vi "GFITS_ExecPreImg.vi"(8 "error in (no error)":errorcluster, 10 "preimg":string="none") -> (0 "error out":errorcluster)   [LabVIEW 2016]
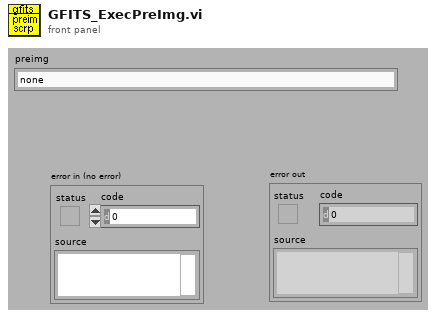
[diagram p1: front panel]
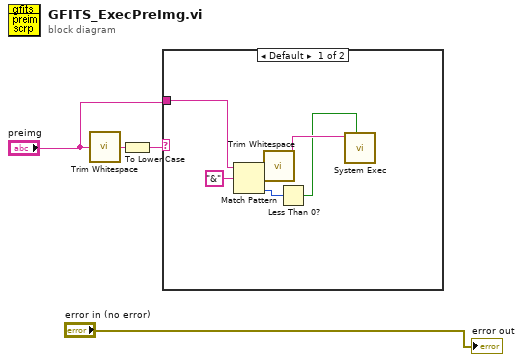
[diagram p0: block diagram]
diagram:
  n1 = call <vilib>:"Trim Whitespace.vi"("string"="preimg") -> ("trimmed string"=w4:string)  [unwired: 1 in]
  n2 = To Lower Case(string=w4) -> (all lower case string=w3:string)
  n3 = case shown="Default" w3 {
    tunnel: "preimg" -> [w10 _]
    frame Default {
      n4 = Match Pattern(string=w10, regular expression="&") -> (before substring=w7:string, offset past match=w8:i32)  [unwired: 3 out]
      n5 = call <vilib>:"Trim Whitespace.vi"("string"=w7) -> ("trimmed string"=w6:string)  [unwired: 1 in]
      n6 = Less Than 0?(x=w8) -> (x < 0?=w5:bool)
      n7 = call <vilib>:"System Exec.vi"("wait until completion? (T)"=w5, "command line"=w6) -> ()  [unwired: 4 in, 6 out]
    }
    frame "", "none" {
    }
  }
  "error out" <- "error in (no error)"
